vi "1,3A PWM MotorControl and VBattSense.vi"() -> ()   [LabVIEW 2011]
doc: "This VI is te Main VI to control the motors and the sense the Battery Voltage.\nMOTORS:\n\nThe motors are limited to given ranges in the setpoint VI. In general, there are two different servos that have to be actuated:\nThe Sailwinch has to work in its full range. The max range of the inout is form 0 to 1. The conversion to PW times is perfromed in Step 2 (In-VI documentation). The maximum range of this Servo was experimentally determined.\nThe Rudder Servo is limited to certain angles. The range of the rudder is determined through the control Rudder Range. The values will be modified by the Rudder Trim control, which allows the user to set a neutral rudder position. \nThe outputs of the Motor control are PWM signal times in us, which are sent to the FPGA VI."
uses:
  2-Think/2 Typedefs/rudder angle.ctl
  2-Think/2 Typedefs/sail setpt.ctl
  <vilib>/FPGAPlugInAG/sbRIO-9606/niLvFpga_Open_sbRIO-9606.vi
  2-Think/2 Globals/2 Global.vi
  <vilib>/Utility/error.llb/Error Cluster From Error Code.vi
  <vilib>/rvi/errors/niLvFpgaAdjustHostInterfaceError.vi
  <vilib>/FPGAPlugInAG/sbRIO-9606/niLvFpga_Close_sbRIO-9606.vi
  <vilib>/rvi/interface/nirviOpenFPGA/nirviOpenFPGA.xnode
  FPGA Bitfiles/SailBot_FPGATarget3_3APWMMotorContro_1677D78E.lvbitx
  FPGA/1,3A PWM-MotorControl and VBattSense FPGA.vi
  <vilib>/rvi/interface/nirviReadWriteControl/nirviReadWriteControl.xnode
  <vilib>/rvi/interface/nirviCloseFPGA/nirviCloseFPGA.xnode
  NiFpgaLv.dll
  FPGA Bitfiles/SailBot_FPGATarget_1,3APWM-MotorCon_DA5FB380.lvbitx
  <vilib>/FPGAPlugInAG/cRIO-9113/niLvFpga_Open_cRIO-9113.vi
panel:
  in  "Reverse Winch Direction":bool=TRUE
  in  "# samples to average":u16=300
  out "Averaged VBatt bitstring":bool[](array[boolean])
  out "vBatt":dbl
  out "vBatt from FPGA\n(unscaled)":u16
  in  "Rudder Range":dbl=80.0
  in  "Rudder Trim":dbl(slide) scale=-20.0..20.0
  out "Sail Position":T1
  out "Rudder Angle":T2
  out "error out":errorcluster
  # "with LSB disabled,\nuncertainty is +-0.08V"
  # "LSB disabled\n(plugged in to \nreserved pin \naccidentally)"
  # "LSB"
  # "MSB"
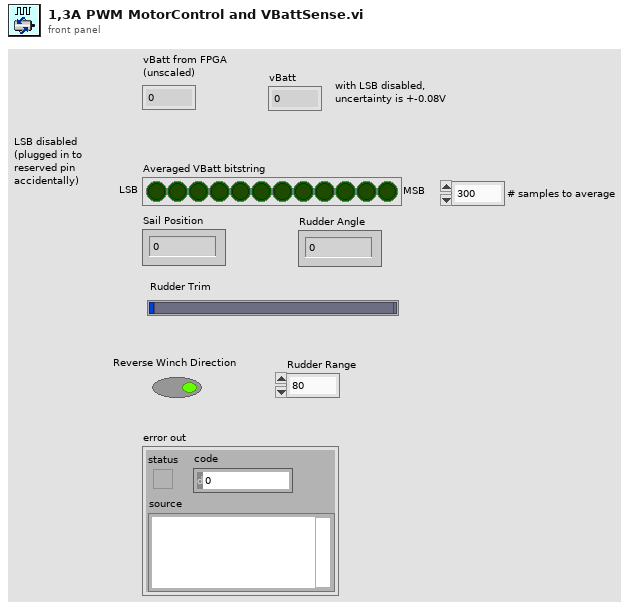
[diagram p1: front panel]
types:
  T1 = typedef "sail setpt.ctl" = dbl
  T2 = typedef "rudder angle.ctl" = dbl
  T3 = typedef "setpoints to boat.ctl" = cluster{"Sail Position":T1, "Rudder Angle":T2}
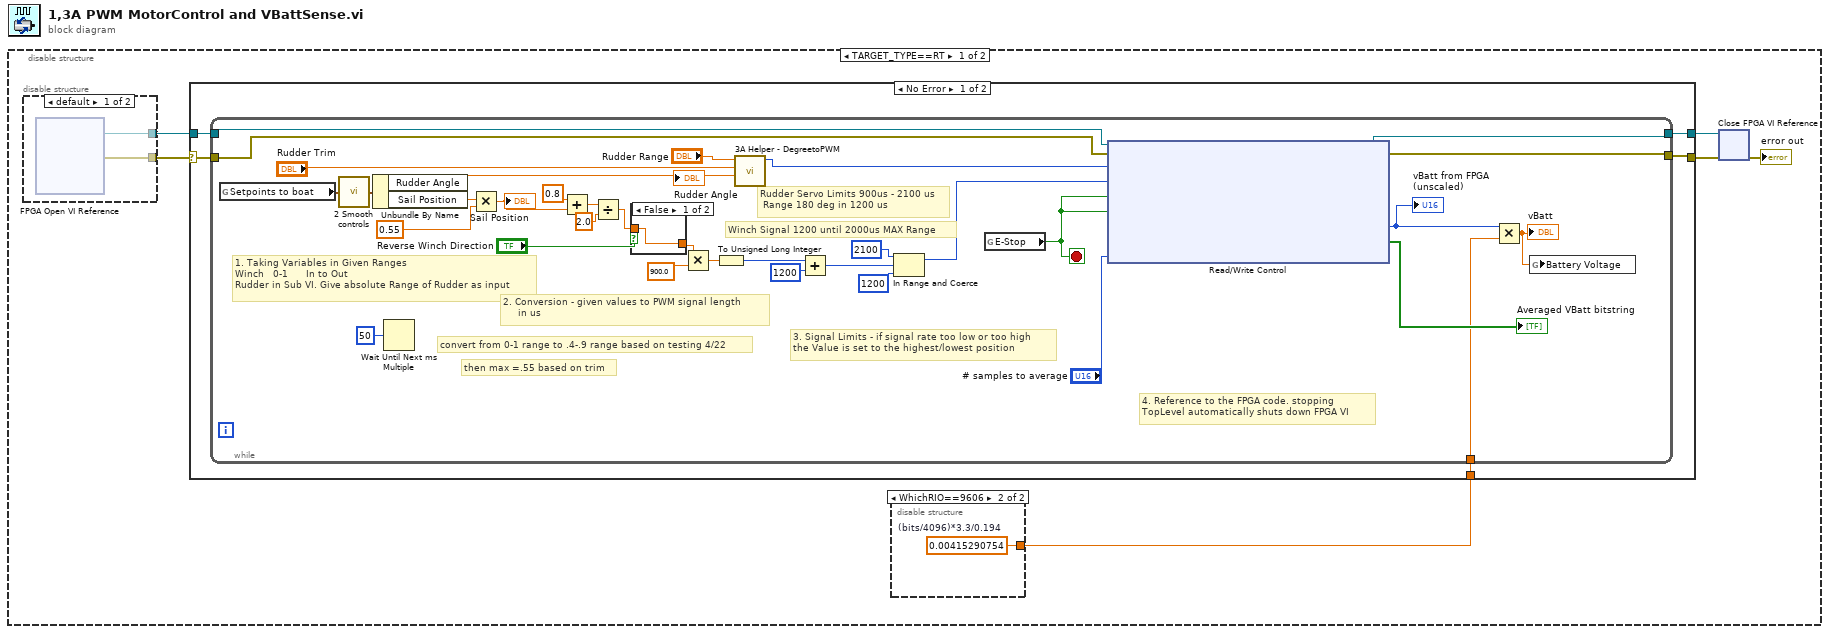
[diagram p0: block diagram]
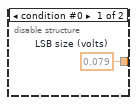
[diagram p2: hidden frame]
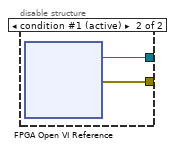
[diagram p3: hidden frame]
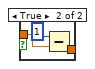
[diagram p4: hidden frame]
diagram:
  n1 = disable-structure shown="TARGET_TYPE==RT" {
    frame condition #0 (active) {
      n2 = disable-structure shown="default" {
        disable-tunnel: [w9 w11] -> w5
        disable-tunnel: [w10 w12] -> w4
        frame condition #0 {
          n3 = xnode "FPGA Open VI Reference"() -> ("FPGA VI Reference Out"=w9:refnum<k20>, "error out"=w10:errorcluster)  [unwired: 2 in]
        }
        frame condition #1 (active) {
          n4 = xnode "FPGA Open VI Reference"() -> ("FPGA VI Reference Out"=w11:refnum<k20>, "error out"=w12:errorcluster)  [unwired: 2 in]
        }
      }
      n5 = disable-structure shown="WhichRIO==9606" {
        disable-tunnel: [w7 w8] -> w1
        frame condition #0 {
          w7 = 0.079  # LSB size (volts)
        }
        frame condition #1 (active) {
          w8 = 0.00415290754  # (bits/4096)*3.3/0.194
        }
      }
      n6 = case shown="No Error" w4 {
        selector: w4 -> [w17 w56]
        tunnel: [w14 w57] -> w3
        tunnel: [w15 w56] -> w2
        tunnel: w5 -> [w16 w57]
        tunnel: w1 -> [w13 _]
        frame No Error {
          n7 = while {
            tunnel: w16 -> [w47]
            tunnel: w17 -> [w48]
            tunnel: [w46] -> w15
            tunnel: [w45] -> w14
            tunnel: w13 -> [w30]
            stop <- w35 stop-if-true
            # "then max =.55 based on trim"
            # "convert from 0-1 range to .4-.9 range based on testing 4/22"
            # "Rudder Servo Limits 900us - 2100 us\n Range 180 deg in 1200 us"
            # "1. Taking Variables in Given Ranges\nWinch   0-1      In to Out\nRudder in Sub VI. Give absolute Range of Rudder as input"
            # "2. Conversion - given values to PWM signal length\n     in us"
            # "3. Signal Limits - if signal rate too low or too high \nthe Value is set to the highest/lowest position"
            # "4. Reference to the FPGA code. stopping \nTopLevel automatically shuts down FPGA VI"
            # "Winch Signal 1200 until 2000us MAX Range"
            n8 = global read "2 Global.vi" "Setpoints to boat"() -> (w19:T3)
            n9 = call "2 Smooth controls.vi"("Setpoints in"=w19) -> ("Smoothed Setpoints out"=w18:T3)  [unwired: 4 in]
            n10 = Unbundle By Name(w18) -> ("Rudder Angle"=w24:T2, "Sail Position"=w22:T1)
            "Rudder Angle" <- w24
            n11 = Wait Until Next ms Multiple(millisecond multiple=u32 50) -> ()  [unwired: 1 out]
            n12 = Multiply(x=w22, y=T1 0.55) -> (x*y=w21:T1)
            "Sail Position" <- w21
            n13 = Add(x=T1 0.8, y=w21) -> (x+y=w26:T1)
            n14 = Divide(x=w26, y=T1 2.0) -> (x/y=w23:T1)
            n15 = case shown="False" "Reverse Winch Direction" {
              tunnel: [w52 w54] -> w29
              tunnel: w23 -> [w52 w53]
              frame False {
              }
              frame True {
                n16 = Subtract(x=1, y=w53) -> (x-y=w54:T1)
              }
            }
            n17 = Multiply(x=w29, y=900.0) -> (x*y=w51:T1)
            n18 = To Unsigned Long Integer(number=w51) -> (unsigned 32bit integer=w50:u32)
            n19 = call "3A Helper - DegreetoPWM.vi"("Rudder Angle"=w24, "Rudder Trim"="Rudder Trim", "Rudder Range (deg)"="Rudder Range") -> ("Servo Position (us)"=w43:u32)  [unwired: 8 in]
            n20 = Add(x=w50, y=u32 1200) -> (x+y=w42:u32)
            n21 = In Range and Coerce(upper limit=u32 2100, x=w42, lower limit=u32 1200) -> (coerced(x)=w39:u32)  [unwired: 1 out]
            n22 = global read "2 Global.vi" "E-Stop"() -> (w35:bool)
            n23 = xnode "Read/Write Control"("FPGA VI Reference In"=w47, "error in"=w48, "Rudder Duty (uSec)"=w43, "Winch Duty (uSec)"=w39, "stop PWM"=w35, "stop VBatt Sense"=w35, "VBatt samples to average"="# samples to average") -> ("FPGA VI Reference Out"=w45:refnum<k20>, "error out"=w46:errorcluster, "vBatt ADC bits"=w34:u16, "Averaged bitstring"=→"Averaged VBatt bitstring":bool[])
            "vBatt from FPGA\n(unscaled)" <- w34
            n24 = Multiply(x=w34, y=w30) -> (x*y=w33:dbl)
            "vBatt" <- w33
            n25 = global write "2 Global.vi" "Battery Voltage"(w33) -> ()
          }
        }
        frame Error {
          # "Error occurred. Do not run."
        }
      }
      n26 = xnode "Close FPGA VI Reference"("FPGA VI Reference In"=w3, "error in"=w2) -> ("error out"=→"error out":errorcluster)
    }
    frame condition #1 {
    }
  }
